vi "Get Index of Child by Tag.vi"(8 "error in (no error)":errorcluster, 10 "Child Tag":string, 11 "Tag Tree In":refnum<class "Tag Tree.lvclass">) -> (0 "error out":errorcluster, 2 "Index":i32, 3 "Tag Tree Out":refnum<class "Tag Tree.lvclass">)   [LabVIEW 2020, in "Tree Helpers.lvlib" / "Tag Tree.lvclass"]
uses:
  Tag Tree.lvclass
  Tag Tree.lvclass/Tag Tree.ctl
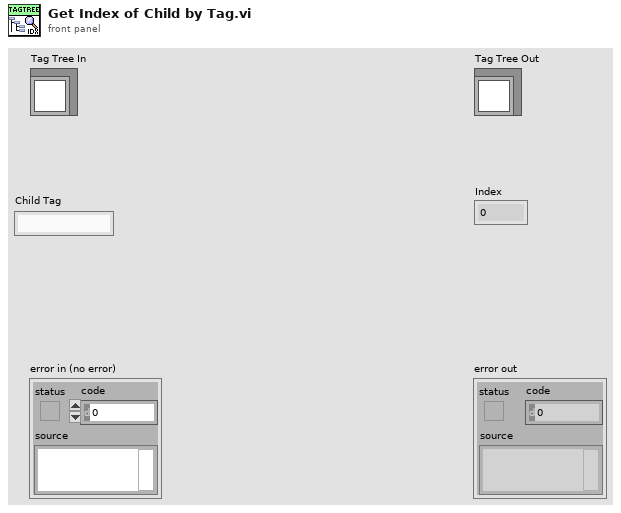
[diagram p1: front panel]
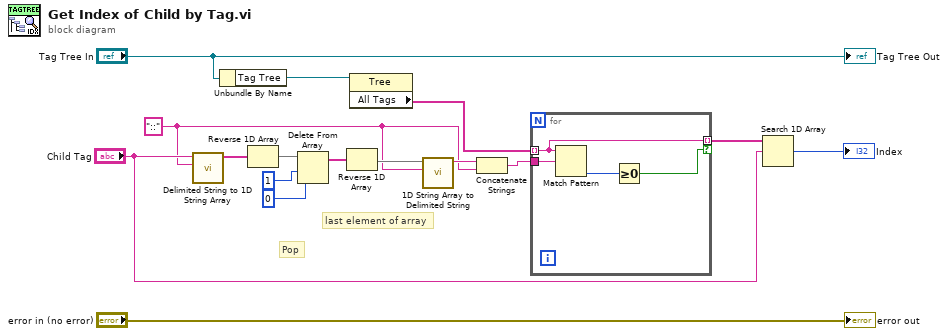
[diagram p0: block diagram]
diagram:
  w1 = "::" ("delimiter")
  # "last element of array"
  # "Pop"
  n1 = call <vilib>:"Delimited String to 1D String Array.vi"("delimiter"=w1, "delimited string"="Child Tag") -> ("string array"=w13:string[])  [unwired: 9 in]
  n2 = Unbundle By Name("Tag Tree In") -> ("Tag Tree"=w14:refnum<vi>)
  n3 = Reverse 1D Array(array=w13) -> (reversed array=w12:string[])
  n4 = Delete From Array(array=w12, length=1, index=0) -> (array with subset deleted=w9:string[])  [unwired: 1 out]
  n5 = Reverse 1D Array(array=w9) -> (reversed array=w8:string[])
  n6 = property class="Tree"(reference=w14) -> ("All Tags"=w7:string[])  [unwired: 1 in, 2 out]
  n7 = call <vilib>:"1D String Array to Delimited String.vi"("delimiter"=w1, "string array"=w8) -> ("delimited string"=w6:string)  [unwired: 9 in]
  n8 = Concatenate Strings(w6, w1) -> (w2:string)
  n9 = for {
    tunnel: w7 -> [w18] mode=indexing
    tunnel: w2 -> [w20]
    tunnel: [w18] -> w5 mode=indexing if=w17
    n10 = Match Pattern(string=w18, regular expression=w20) -> (offset past match=w19:i32)  [unwired: 1 in, 3 out]
    n11 = Greater Or Equal To 0?(x=w19) -> (x >= 0?=w17:bool)
  }
  n12 = Search 1D Array(1D array=w5, element="Child Tag") -> (index of element=→"Index":i32)  [unwired: 1 in]
  "error out" <- "error in (no error)"
  "Tag Tree Out" <- "Tag Tree In"
